vi "DAQmx.Get Calibration.vi"(8 "error in (no error)":errorcluster, 11 "DAQmx in":refnum<class "DAQmx.lvclass">) -> (0 "error out":errorcluster, 2 "Calibration out":T1(array[cluster]), 3 "DAQmx out":refnum<class "DAQmx.lvclass">)   [LabVIEW 2019, in "DAQmx.lvclass"]
uses:
  DAQmx.lvclass
  DAQmx.lvclass/DAQmx.ctl
  <resource>/objmgr/daqmx.rc
panel:
  out "cal due?":bool
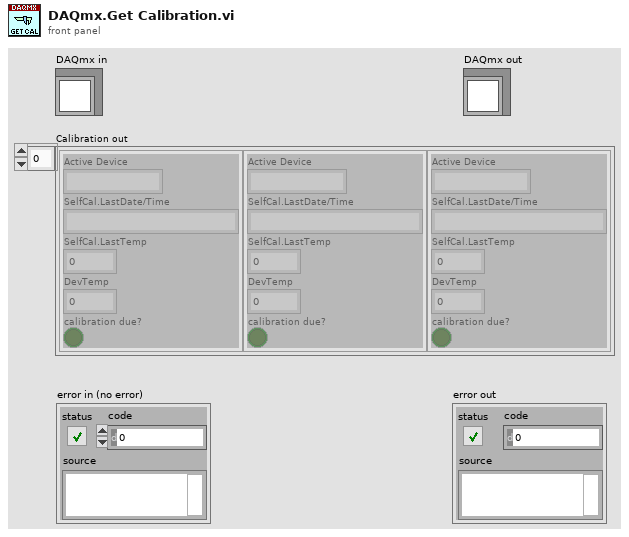
[diagram p1: front panel]
types:
  T1 = cluster{"Active Device":string, "SelfCal.LastDate/Time":string, "SelfCal.LastTemp":dbl, "DevTemp":dbl, "calibration due?":bool}[]
  T2 = cluster{"Active Device":string, "SelfCal.LastDate/Time":string, "SelfCal.LastTemp":dbl, "DevTemp":dbl, "calibration due?":bool}
  T3 = typedef "DAQmx.lvclass/DeviceInfo--Cluster.ctl" = cluster{"DeviceName":string, "DevIsSimulated":bool, "DeviceSerialNumber":string, "ProductType":string, "ProductCategory":i32, "ProductNumber":u32, "ChassisNumber":u32, "SlotNumber":u32, "ChassisName":string, "ChassisSerialNumber":string, "DevTemp":dbl, "SelfCal.LastDate/Time":string, "SelfCal.LastTemp":dbl, "calibration due?":bool}
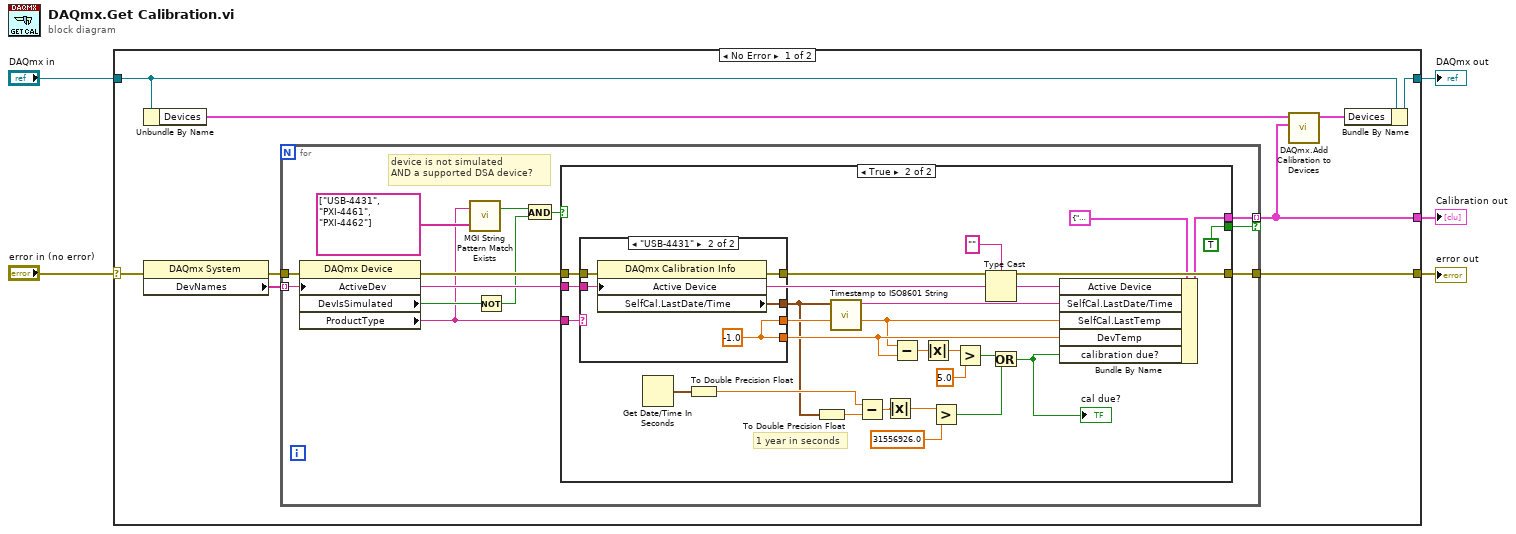
[diagram p0: block diagram]
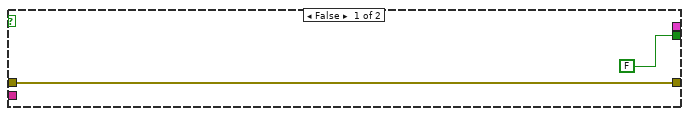
[diagram p2: hidden frame]
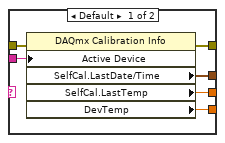
[diagram p3: hidden frame]
diagram:
  n1 = case shown="No Error" "error in (no error)" {
    selector: "error in (no error)" -> [w11 w65]
    tunnel: [w9 w65] -> w5
    tunnel: "DAQmx in" -> [w10 w66]
    tunnel: [w14 w66] -> w3
    tunnel: [w6 _] -> w1
    frame No Error {
      n2 = Unbundle By Name(w10) -> ("Devices"=w8:T3[])
      n3 = property class="DAQmx System"(error in=w11) -> (error out=w12:errorcluster, "DevNames"=w13:tag[])  [unwired: 1 in, 1 out]
      n4 = for {
        tunnel: w13 -> [w24] mode=indexing
        tunnel: w12 -> [w25]
        tunnel: [w26] -> w9
        tunnel: [w19] -> w6 mode=indexing if=w18
        # "device is not simulated\nAND a supported DSA device?"
        n5 = property class="DAQmx Device"(error in=w25, "ActiveDev"=w24) -> (error out=w23:errorcluster, "DevIsSimulated"=w22:bool, "ProductType"=w17:string)  [unwired: 1 in, 1 out]
        n6 = call <userlib>:"MGI String Pattern Match Exists.vi"("Patterns to Try"=string[] ["USB-4431", "PXI-4461", "PXI-4462"], "String"=w17) -> ("Match Found"=w15:bool)  [unwired: 1 out]
        n7 = Not(x=w22) -> (.not. x?=w16:bool)
        n8 = And(x=w15, y=w16) -> (x .and. y?=w21:bool)
        n9 = case shown="True" w21 {
          tunnel: [w28 w53] -> w26
          tunnel: w24 -> [_ w42]
          tunnel: w23 -> [w28 w41]
          tunnel: [FALSE TRUE] -> w18
          tunnel: [_ w30] -> w19
          tunnel: w17 -> [_ w29]
          frame False {
          }
          frame True {
            # "1 year in seconds"
            n10 = case shown="\"USB-4431\"" w29 {
              tunnel: [w59 w64] -> w53
              tunnel: [w58 w60] -> w49
              tunnel: [w57 w60] -> w48
              tunnel: w42 -> [w56 w63]
              tunnel: w41 -> [w55 w62]
              tunnel: [w54 w61] -> w33
              frame Default {
                n11 = property class="DAQmx Calibration Info"(error in=w55, "Active Device"=w56) -> (error out=w59:errorcluster, "SelfCal.LastDate/Time"=w54:timestamp, "SelfCal.LastTemp"=w57:dbl, "DevTemp"=w58:dbl)  [unwired: 1 in, 1 out]
              }
              frame "USB-4431" {
                w60 = -1.0 ("DevTemp")
                n12 = property class="DAQmx Calibration Info"(error in=w62, "Active Device"=w63) -> (error out=w64:errorcluster, "SelfCal.LastDate/Time"=w61:timestamp)  [unwired: 1 in, 1 out]
              }
            }
            n13 = Get Date/Time In Seconds() -> (seconds since 1Jan1904=w38:timestamp)
            n14 = To Double Precision Float(number=w38) -> (double precision float=w36:dbl)
            n15 = To Double Precision Float(number=w33) -> (double precision float=w37:dbl)
            n16 = call <vilib>:"Timestamp to ISO8601 String.vi"("Timestamp (now)"=w33) -> ("ISO8601 String"=w32:string)  [unwired: 10 in]
            n17 = Subtract(x=w36, y=w37) -> (x-y=w47:dbl)
            n18 = Absolute Value(x=w47) -> (abs(x)=w46:dbl)
            n19 = Subtract(x=w48, y=w49) -> (x-y=w52:dbl)
            n20 = Absolute Value(x=w52) -> (abs(x)=w51:dbl)
            n21 = Greater?(x=w46, y=31556926.0) -> (0:w44:bool)
            n22 = Greater?(x=w51, y=5.0) -> (0:w45:bool)
            n23 = Type Cast(type="", x=w42) -> (*(type *) &x=w35:string)
            n24 = Or(x=w45, y=w44) -> (x .or. y?=w39:bool)
            "cal due?" <- w39
            n25 = Bundle By Name(cluster=T2 {"Active Device"="", "SelfCal.LastDate/Time"="", "SelfCal.LastTemp"=0.0, "DevTemp"=0.0, "calibration due?"=FALSE} ("element"), "Active Device"=w35, "SelfCal.LastDate/Time"=w32, "SelfCal.LastTemp"=w48, "DevTemp"=w49, "calibration due?"=w39) -> (w30:T2)
          }
        }
      }
      n26 = call "DAQmx.Add Calibration to Devices.vi"("Calibration in"=w6, "Devices in"=w8) -> ("Devices out"=w7:T3[])  [unwired: 9 in]
      n27 = Bundle By Name(cluster=w10, "Devices"=w7) -> (w14:refnum<class "DAQmx.lvclass">)
    }
    frame Error {
    }
  }
  "error out" <- w5
  "Calibration out" <- w1
  "DAQmx out" <- w3
